vi "(SubVI) Delete xDNA and Force is negative or positive.vi"(3 "xDNA":dbl[](array[numeric]), 4 "T=positive (RHS)\nF=negative (LHS)":bool, 5 "Force":dbl[](array[numeric])) -> (0 "xDNA-cut":dbl[](array[numeric]), 2 "Force-cut":dbl[](array[numeric]))   [LabVIEW 2014]
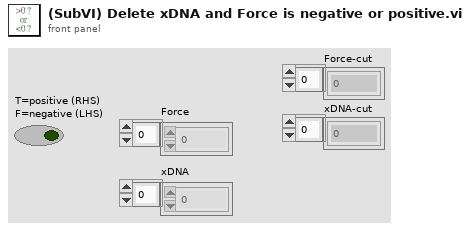
[diagram p1: front panel]
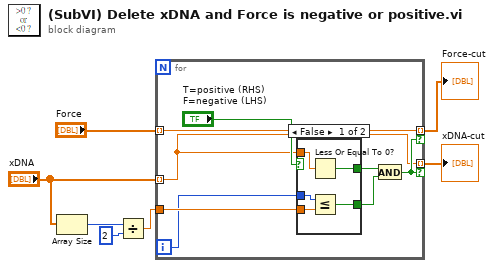
[diagram p0: block diagram]
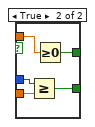
[diagram p2: hidden frame]
diagram:
  n1 = Array Size(array="xDNA") -> (size(s)=w5:i32)
  n2 = Divide(x=w5, y=2) -> (x/y=w3:dbl)
  n3 = for {
    tunnel: [w14] -> w7 mode=indexing if=w10
    tunnel: "Force" -> [w14] mode=indexing
    tunnel: [w9] -> w6 mode=indexing if=w10
    tunnel: "xDNA" -> [w9] mode=indexing
    tunnel: w3 -> [w12]
    i -> [w8]
    n4 = case shown="False" "T=positive (RHS)\nF=negative (LHS)" {
      tunnel: [w20 w25] -> w13
      tunnel: w8 -> [w18 w24]
      tunnel: w12 -> [w17 w23]
      tunnel: [w19 w22] -> w11
      tunnel: w9 -> [w16 w21]
      frame False {
        n5 = Less Or Equal To 0?(x=w16) -> (x <= 0?=w20:bool)
        n6 = Less Or Equal?(x=w18, y=w17) -> (x <= y?=w19:bool)
      }
      frame True {
        n7 = Greater Or Equal?(x=w24, y=w23) -> (x >= y?=w22:bool)
        n8 = Greater Or Equal To 0?(x=w21) -> (x >= 0?=w25:bool)
      }
    }
    n9 = And(x=w13, y=w11) -> (x .and. y?=w10:bool)
  }
  "Force-cut" <- w7
  "xDNA-cut" <- w6
